vi "频谱.vi"() -> ()   [LabVIEW 2010]
uses:
  <vilib>/express/express analysis/Spectral/XNode/ExpressSpectralMeasurementsBlockNode.xnode
  Instance           4 12Saved   频谱 .vi
  Instance           6 12Saved   频谱 .vi
  Instance           1 12Saved   频谱 .vi
  Instance           5 12Saved   频谱 .vi
  Instance           8 12Saved   频谱 .vi
  Instance           2 12Saved   频谱 .vi
  <vilib>/express/express analysis/Spectral/Block/exnSpectralBlock spectral measurements peak poly.vi
  <vilib>/express/express analysis/Spectral/Block/exnSpectralBlock spectral measurements peak DDT.vi
panel:
  in  "增益":dbl
  out "温度计":dbl(slide) scale=0.0..100.0
  in  "低端截止频率":dbl
  in  "选择轴承":i32
  out "频谱":dbl[](graph)
  in  "滤波器开":bool
  out "波形图":dynamicdata(graph)
  in  "stop (F)":bool
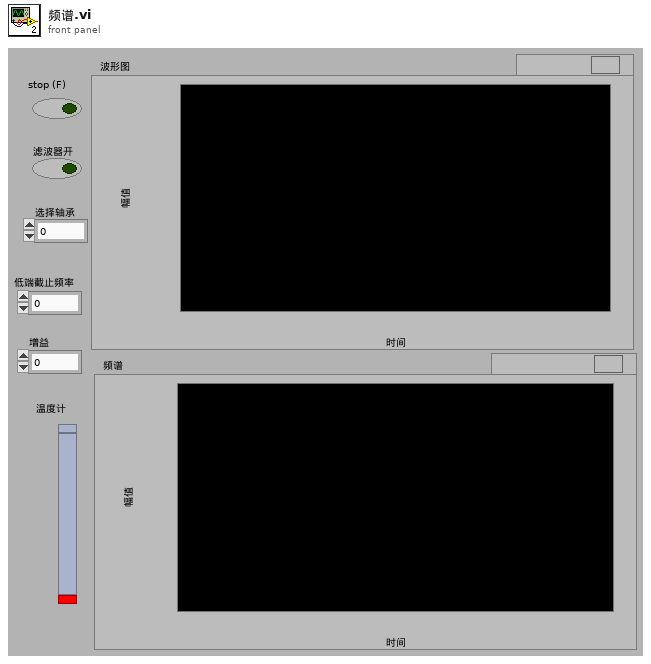
[diagram p1: front panel]
types:
  T1 = cluster{"averaging mode":u16, "weighting mode":u16, "number of averages":u32}
  T2 = cluster{"dB On (F)":bool, "unwrap phase (F)":bool, "convert to degree (F)":bool}
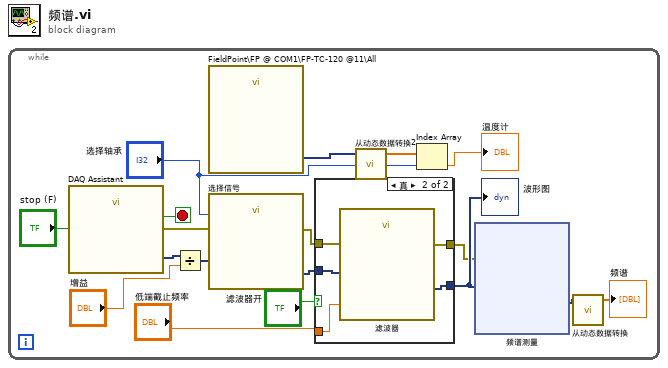
[diagram p0: block diagram]
diagram:
  n1 = while {
    stop <- w17 stop-if-true
    n2 = call "DAQ Assistant"("stop (F)"="stop (F)") -> ("data"=w14:dynamicdata, "stopped"=w17:bool, "error out"=w10:errorcluster)  [unwired: 15 in, 1 out]
    n3 = Divide(x=w14, y="增益") -> (x/y=w2:dynamicdata)
    n4 = call "FieldPoint\\FP @ COM1\\FP-TC-120 @11\\All"() -> ("Value out"=w6:dynamicdata)  [unwired: 5 in, 2 out]
    n5 = call "选择信号"("error in (no error)"=w10, "Selector Input"="选择轴承", "Signals"=w2) -> ("error out"=w9:errorcluster, "Signal Out"=w13:dynamicdata)  [unwired: 7 in]
    n6 = case shown="真" "滤波器开" {
      tunnel: w13 -> [w30 w35]
      tunnel: [w30 w34] -> w12
      tunnel: w9 -> [w29 w33]
      tunnel: [w29 w32] -> w8
      tunnel: "低端截止频率" -> [_ w31]
      frame False {
      }
      frame True {
        n7 = call "滤波器"("error in (no error)"=w33, "Lower Cut-Off"=w31, "Signal"=w35) -> ("error out"=w32:errorcluster, "Filtered Signal"=w34:dynamicdata)  [unwired: 7 in]
      }
    }
    "波形图" <- w12
    n8 = call "从动态数据转换2"("Dynamic Data Type"=w6) -> ("Array"=w5:dbl[])  [unwired: 3 in]
    n9 = Index Array(array=w5, index="选择轴承") -> (element=→"温度计":dbl)
    n10 = xnode "频谱测量"("信号"=w12, "错误输入（无错误）"=w8) -> ("FFT - （峰值）"=w15:dynamicdata)  [unwired: 2 out]
    n11 = call "从动态数据转换"("Dynamic Data Type"=w15) -> ("Array"=→"频谱":dbl[])  [unwired: 3 in]
  }
